vi "LLB - By List.vi"(7 "Msg Chain":string, 8 "error in (no error)":errorcluster {"code" format="Error %.0f"}, 10 "LLBs":refnum<class "LLB Documentation.lvclass">[](array[class]), 11 "VIDoc Printer - Confluence In":refnum<class "VIDoc Printer - Confluence.lvclass">) -> (0 "error out":errorcluster {"code" format="Error %.0f"}, 3 "VIDoc Printer - Confluence Out":refnum<class "VIDoc Printer - Confluence.lvclass">)   [LabVIEW 2023, in "VIDoc Printer - Confluence.lvlib" / "VIDoc Printer - Confluence.lvclass"]
uses:
  VIDoc Printer - Confluence.lvclass
  Parsing/LLB Documentation/LLB Documentation.lvclass
  VIDoc Printer - Confluence.lvclass/VIDoc Printer - Confluence.ctl
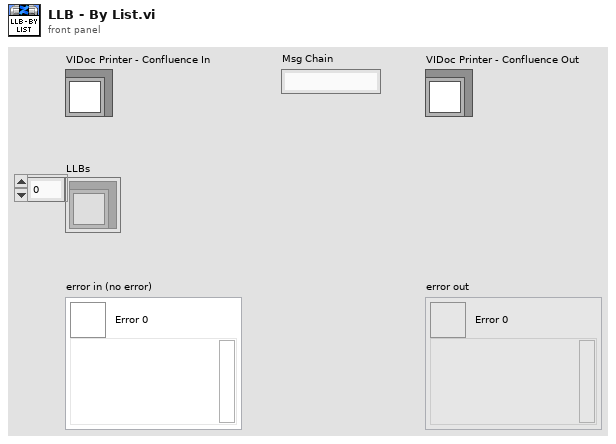
[diagram p1: front panel]
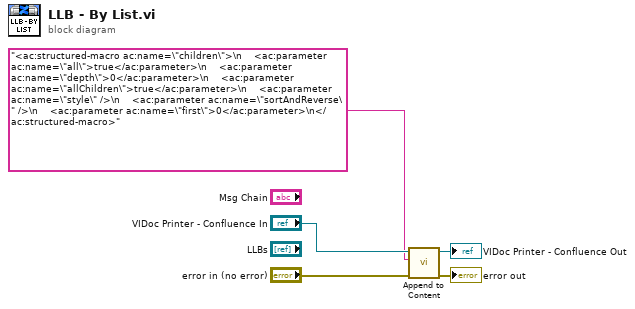
[diagram p0: block diagram]
diagram:
  n1 = call "Append to Content.vi"("error in (no error)"="error in (no error)", "Content"="<ac:structured-macro ac:name=\"children\">\n    <ac:parameter ac:name=\"all\">true</ac:parameter>\n    <ac:parameter ac:name=\"depth\">0</ac:parameter>\n    <ac:parameter ac:name=\"allChildren\">true</ac:parameter>\n    <ac:parameter ac:name=\"style\" />\n    <ac:parameter ac:name=\"sortAndReverse\" />\n    <ac:parameter ac:name=\"first\">0</ac:parameter>\n</ac:structured-macro>", "Confluence Printer in"="VIDoc Printer - Confluence In") -> ("error out"=→"error out":errorcluster, "Confluence Printer out"=→"VIDoc Printer - Confluence Out":refnum<class "VIDoc Printer - Confluence.lvclass">)  [unwired: 7 in]
